vi "Read TCP Message - Prepended Size Version.vi"(7 "Server Alias":string, 8 "Error In":errorcluster, 11 "TCP Connection In":refnum<k5>) -> (0 "Error Out":errorcluster, 2 "Data Read":string, 3 "TCP Connection Out":refnum<k5>, 4 "Message Length":i32)   [LabVIEW 2013, in "TS.lvlib"]
uses:
  TS.lvlib
panel:
  out "Size in Bytes":string
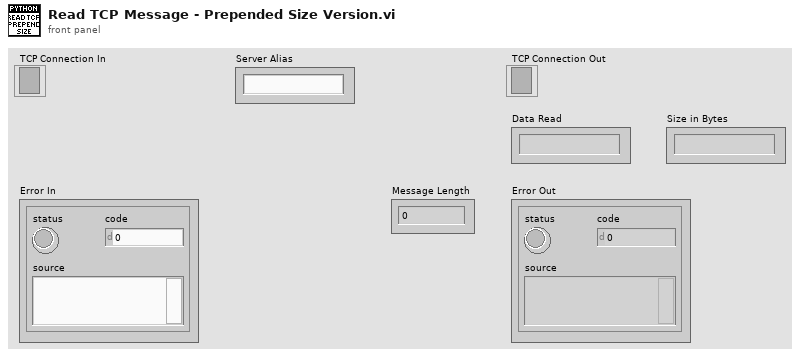
[diagram p1: front panel]
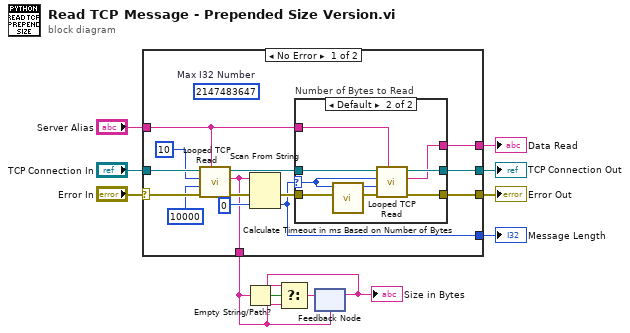
[diagram p0: block diagram]
diagram:
  n1 = case shown="No Error" "Error In" {
    selector: "Error In" -> [w25 w37]
    tunnel: "TCP Connection In" -> [w24 w36]
    tunnel: [w20 w37] -> w9
    tunnel: [w21 w36] -> w8
    tunnel: [w19 _] -> w7
    tunnel: [w14 _] -> w4
    tunnel: [w13 _] -> w2
    tunnel: "Server Alias" -> [w12 _]
    frame No Error {
      (unwired) 2147483647  # Max I32 Number
      n2 = call "Looped TCP Read.vi"("Server Alias"=w12, "error in (no error)"=w25, "timeout ms (25000)"=10000, "bytes to read"=10, "connection ID in"=w24) -> ("error out"=w17:errorcluster, "data out"=w14:string, "connection ID out"=w22:refnum<k5>)  [unwired: 4 in]
      n3 = Scan From String(input string=w14, error in=w17, default 1=0 ("bytes to read")) -> (error out=w16:errorcluster, output 1=w13:i32)  [unwired: 2 in, 2 out]
      n4 = case "Number of Bytes to Read" shown="Default" w13 {
        selector: w13 -> [_ w30]
        tunnel: w22 -> [w27 w35]
        tunnel: w16 -> [w26 w34]
        tunnel: [w27 w33] -> w21
        tunnel: [w26 w32] -> w20
        tunnel: [_ w31] -> w19
        tunnel: w12 -> [_ w28]
        frame ..0 {
          # "No data."
        }
        frame Default {
          n5 = call "Calculate Timeout in ms Based on Number of Bytes.vi"("Number of Bytes"=w30) -> ("Timeout (ms)"=w29:i32)  [unwired: 10 in]
          n6 = call "Looped TCP Read.vi"("Server Alias"=w28, "error in (no error)"=w34, "timeout ms (25000)"=w29, "bytes to read"=w30, "connection ID in"=w35) -> ("error out"=w32:errorcluster, "data out"=w31:string, "connection ID out"=w33:refnum<k5>)  [unwired: 4 in]
        }
      }
    }
    frame Error {
    }
  }
  "Error Out" <- w9
  "TCP Connection Out" <- w8
  "Data Read" <- w7
  "Message Length" <- w2
  n7 = Empty String/Path?(string/path=w4) -> (empty?=w5:bool)
  n8 = feedback #1(w4) -> (w3:string)
  "Size in Bytes" <- w3
  n9 = Select(t=w3, s=w5, f=w4) -> (s? t:f=w6:string)
  n10 = feedback-in #1(w6) -> ()
